vi "Example Data Thing.vi"() -> ()   [LabVIEW 2018]
uses:
  <vilib>/Utility/miscctls.llb/LVForegroundBackgroundColorsTypeDef.ctl
panel:
  in  "Hammertime":bool
  in  "Numeric":dbl format="%#_13g"
  out "Gyro":dbl(knob) scale=0.0..360.0
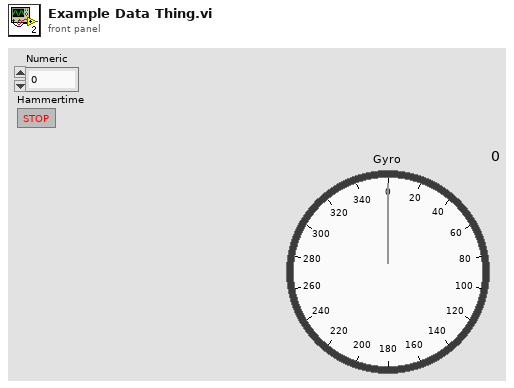
[diagram p1: front panel]
types:
  T1 = typedef "LVForegroundBackgroundColorsTypeDef.ctl" = cluster{"Foreground Color":u32, "Background Color":u32}
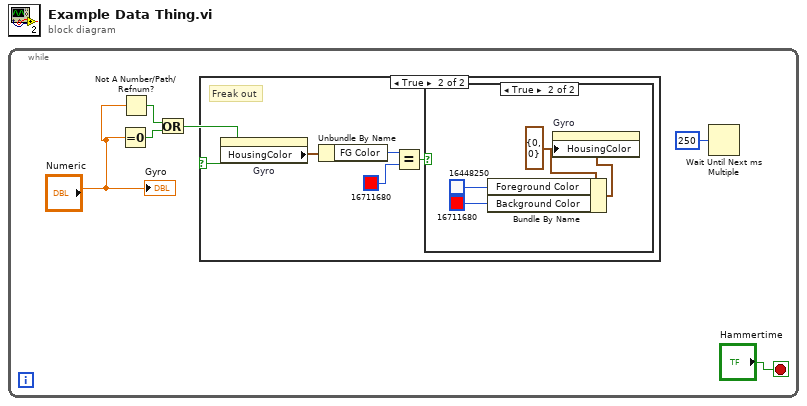
[diagram p0: block diagram]
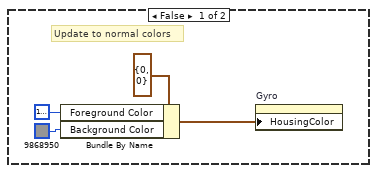
[diagram p2: hidden frame]
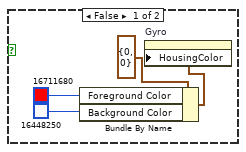
[diagram p3: hidden frame]
diagram:
  n1 = while {
    stop <- "Hammertime" stop-if-true
    n2 = Equal To 0?(x="Numeric") -> (x = 0?=w2:bool)
    n3 = Not A Number/Path/Refnum?(number/path/refnum="Numeric") -> (NaN/Path/Refnum?=w3:bool)
    n4 = Or(x=w3, y=w2) -> (x .or. y?=w1:bool)
    n5 = case shown="True" w1 {
      frame False {
        # "Update to normal colors"
        n6 = Bundle By Name(cluster=T1 {"Foreground Color"=0, "Background Color"=0} ("Housing Colors"), "Foreground Color"=u32 16777222, "Background Color"=u32 9868950) -> (w10:T1)
        n7 = property on="Gyro" class="Knob (strict)"("HousingColor"=w10) -> ()  [unwired: 2 in, 2 out]
      }
      frame True {
        # "Freak out"
        n8 = property on="Gyro" class="Knob (strict)"() -> ("HousingColor"=w14:T1)  [unwired: 2 in, 2 out]
        n9 = Unbundle By Name(w14) -> ("FG Color"=w13:u32)
        n10 = Equal?(x=w13, y=u32 16711680) -> (x = y?=w11:bool)
        n11 = case shown="True" w11 {
          frame False {
            n12 = Bundle By Name(cluster=T1 {"Foreground Color"=0, "Background Color"=0} ("Housing Colors"), "Foreground Color"=u32 16711680, "Background Color"=u32 16448250) -> (w17:T1)
            n13 = property on="Gyro" class="Knob (strict)"("HousingColor"=w17) -> ()  [unwired: 2 in, 2 out]
          }
          frame True {
            n14 = Bundle By Name(cluster=T1 {"Foreground Color"=0, "Background Color"=0} ("Housing Colors"), "Foreground Color"=u32 16448250, "Background Color"=u32 16711680) -> (w22:T1)
            n15 = property on="Gyro" class="Knob (strict)"("HousingColor"=w22) -> ()  [unwired: 2 in, 2 out]
          }
        }
      }
    }
    n16 = Wait Until Next ms Multiple(millisecond multiple=u32 250) -> ()  [unwired: 1 out]
    "Gyro" <- "Numeric"
  }
